vi "Game Engine.vi"(6 "UI Refs":T1, 10 "Dashboard":T2[](array[typedef]), 11 "SquareBattle in":refnum<class "SquareBattle.lvclass">) -> ()   [LabVIEW 2014, in "SquareBattle.lvclass"]
uses:
  SquareBattle.lvclass
  Dashboard.ctl
  UI Refs.ctl
  Runner Cluster.ctl
  Runner/Runner.lvclass
  Move State Cluster.ctl
  Action Enum.ctl
  Move Queue Element Cluster.ctl
  Direction Enum.ctl
  SquareBattle.lvclass/SquareBattle.ctl
  Runner/Runner.lvclass/Runner.ctl
panel:
  # "NOTICE - YOU MUST NOT REMOVE THIS NOTICE. PER THE FOLLOWING LICENSE, YOU MAY REPRODUCE THIS SOFTWARE PROVIDED YOU FOLLOW THE TERMS\nOF THE LICENSE.\n\n---BEGIN BSD LICENSE (http://opensource.org/licenses/BSD-2-Clause)---\nCopyright (c) 2015, Endigit, Inc. <robert@endigit.com>\nAll rights reserved.\n\nRedistribution and use in source and binary forms, with or without modification, are permitted provided that the following conditions are met:\n\n1. Redistributions of source code must retain the above copyright notice, this list of conditions and the following disclaimer.\n\n2. Redistributions in binary form must reproduce the above copyright notice, this list of conditions and the following disclaimer in the documentation and/or other \nmaterials provided with the distribution.\n\nTHIS SOFTWARE IS PROVIDED BY THE COPYRIGHT HOLDERS AND CONTRIBUTORS \"AS IS\" AND ANY EXPRESS OR IMPLIED WARRANTIES, INCLUDING, BUT NOT \nLIMITED TO, THE IMPLIED WARRANTIES OF MERCHANTABILITY AND FITNESS FOR A PARTICULAR PURPOSE ARE DISCLAIMED. IN NO EVENT SHALL THE COPYRIGHT \nHOLDER OR CONTRIBUTORS BE LIABLE FOR ANY DIRECT, INDIRECT, INCIDENTAL, SPECIAL, EXEMPLARY, OR CONSEQUENTIAL DAMAGES (INCLUDING, BUT NOT \nLIMITED TO, PROCUREMENT OF SUBSTITUTE GOODS OR SERVICES; LOSS OF USE, DATA, OR PROFITS; OR BUSINESS INTERRUPTION) HOWEVER CAUSED AND ON \nANY THEORY OF LIABILITY, WHETHER IN CONTRACT, STRICT LIABILITY, OR TORT (INCLUDING NEGLIGENCE OR OTHERWISE) ARISING IN ANY WAY OUT OF THE USE \nOF THIS SOFTWARE, EVEN IF ADVISED OF THE POSSIBILITY OF SUCH DAMAGE.\n---END BSD LICENSE---"
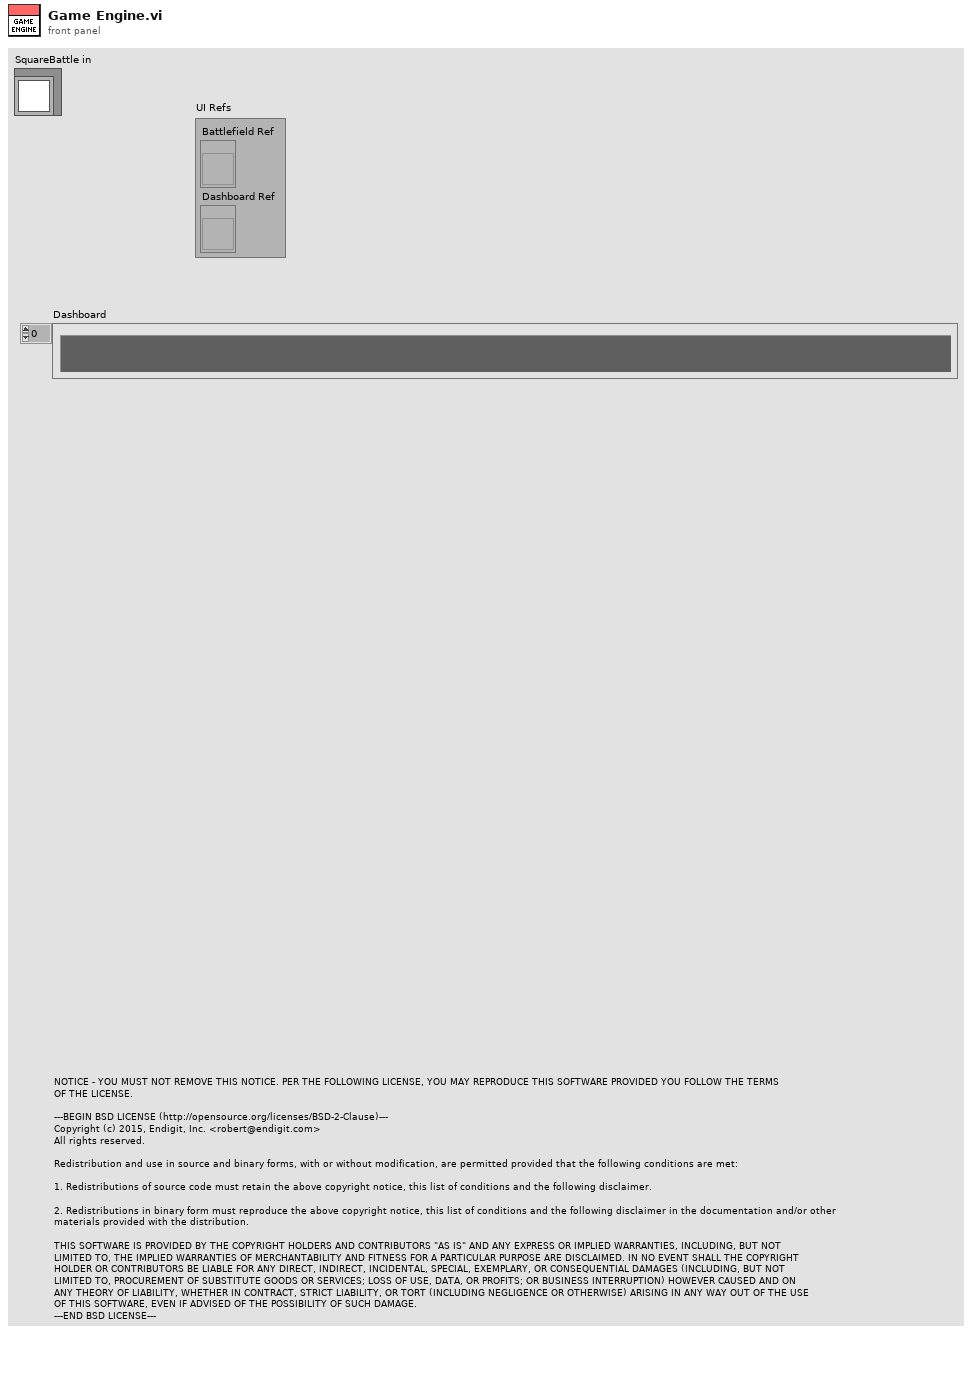
[diagram p1: front panel]
types:
  T1 = typedef "SquareBattle.lvclass/UI Refs.ctl" = cluster{"Battlefield Ref":refnum<vi>, "Dashboard Ref":refnum<vi>}
  T2 = typedef "SquareBattle.lvclass/Dashboard.ctl" = cluster{"Color":u32, "Player":string, "Status":string}
  T3 = typedef "SquareBattle.lvclass/Move Queue Element Cluster.ctl" = cluster{"Team Idx":i32, "NextTurn":u32, "YX Pos":string, "s Taken":dbl, "RunnerRef":refnum<data-value>, "Action":T4, "Direction":T5, "Player#":i32, "Replicated":refnum<class "Runner.lvclass">}
  T4 = typedef "SquareBattle.lvclass/Action Enum.ctl" = enum16{"Wait", "Move", "Attack", "Replicate"}
  T5 = typedef "SquareBattle.lvclass/Direction Enum.ctl" = enum16{"NW", "N", "NE", "E", "SE", "S", "SW", "W"}
  T6 = typedef "SquareBattle.lvclass/Move State Cluster.ctl" = cluster{"InPlayPos Dict":variant}
  T7 = typedef "SquareBattle.lvclass/Runner Cluster.ctl" = cluster{"Attacked?":bool, "DVR":refnum<data-value>, "Team":i32, "Player":i32, "Wait":u32}
  T8 = typedef "SquareBattle.lvclass/Player Info.ctl" = cluster{"Name":string, "Color Box":u32, "Gloat Phrase":string}
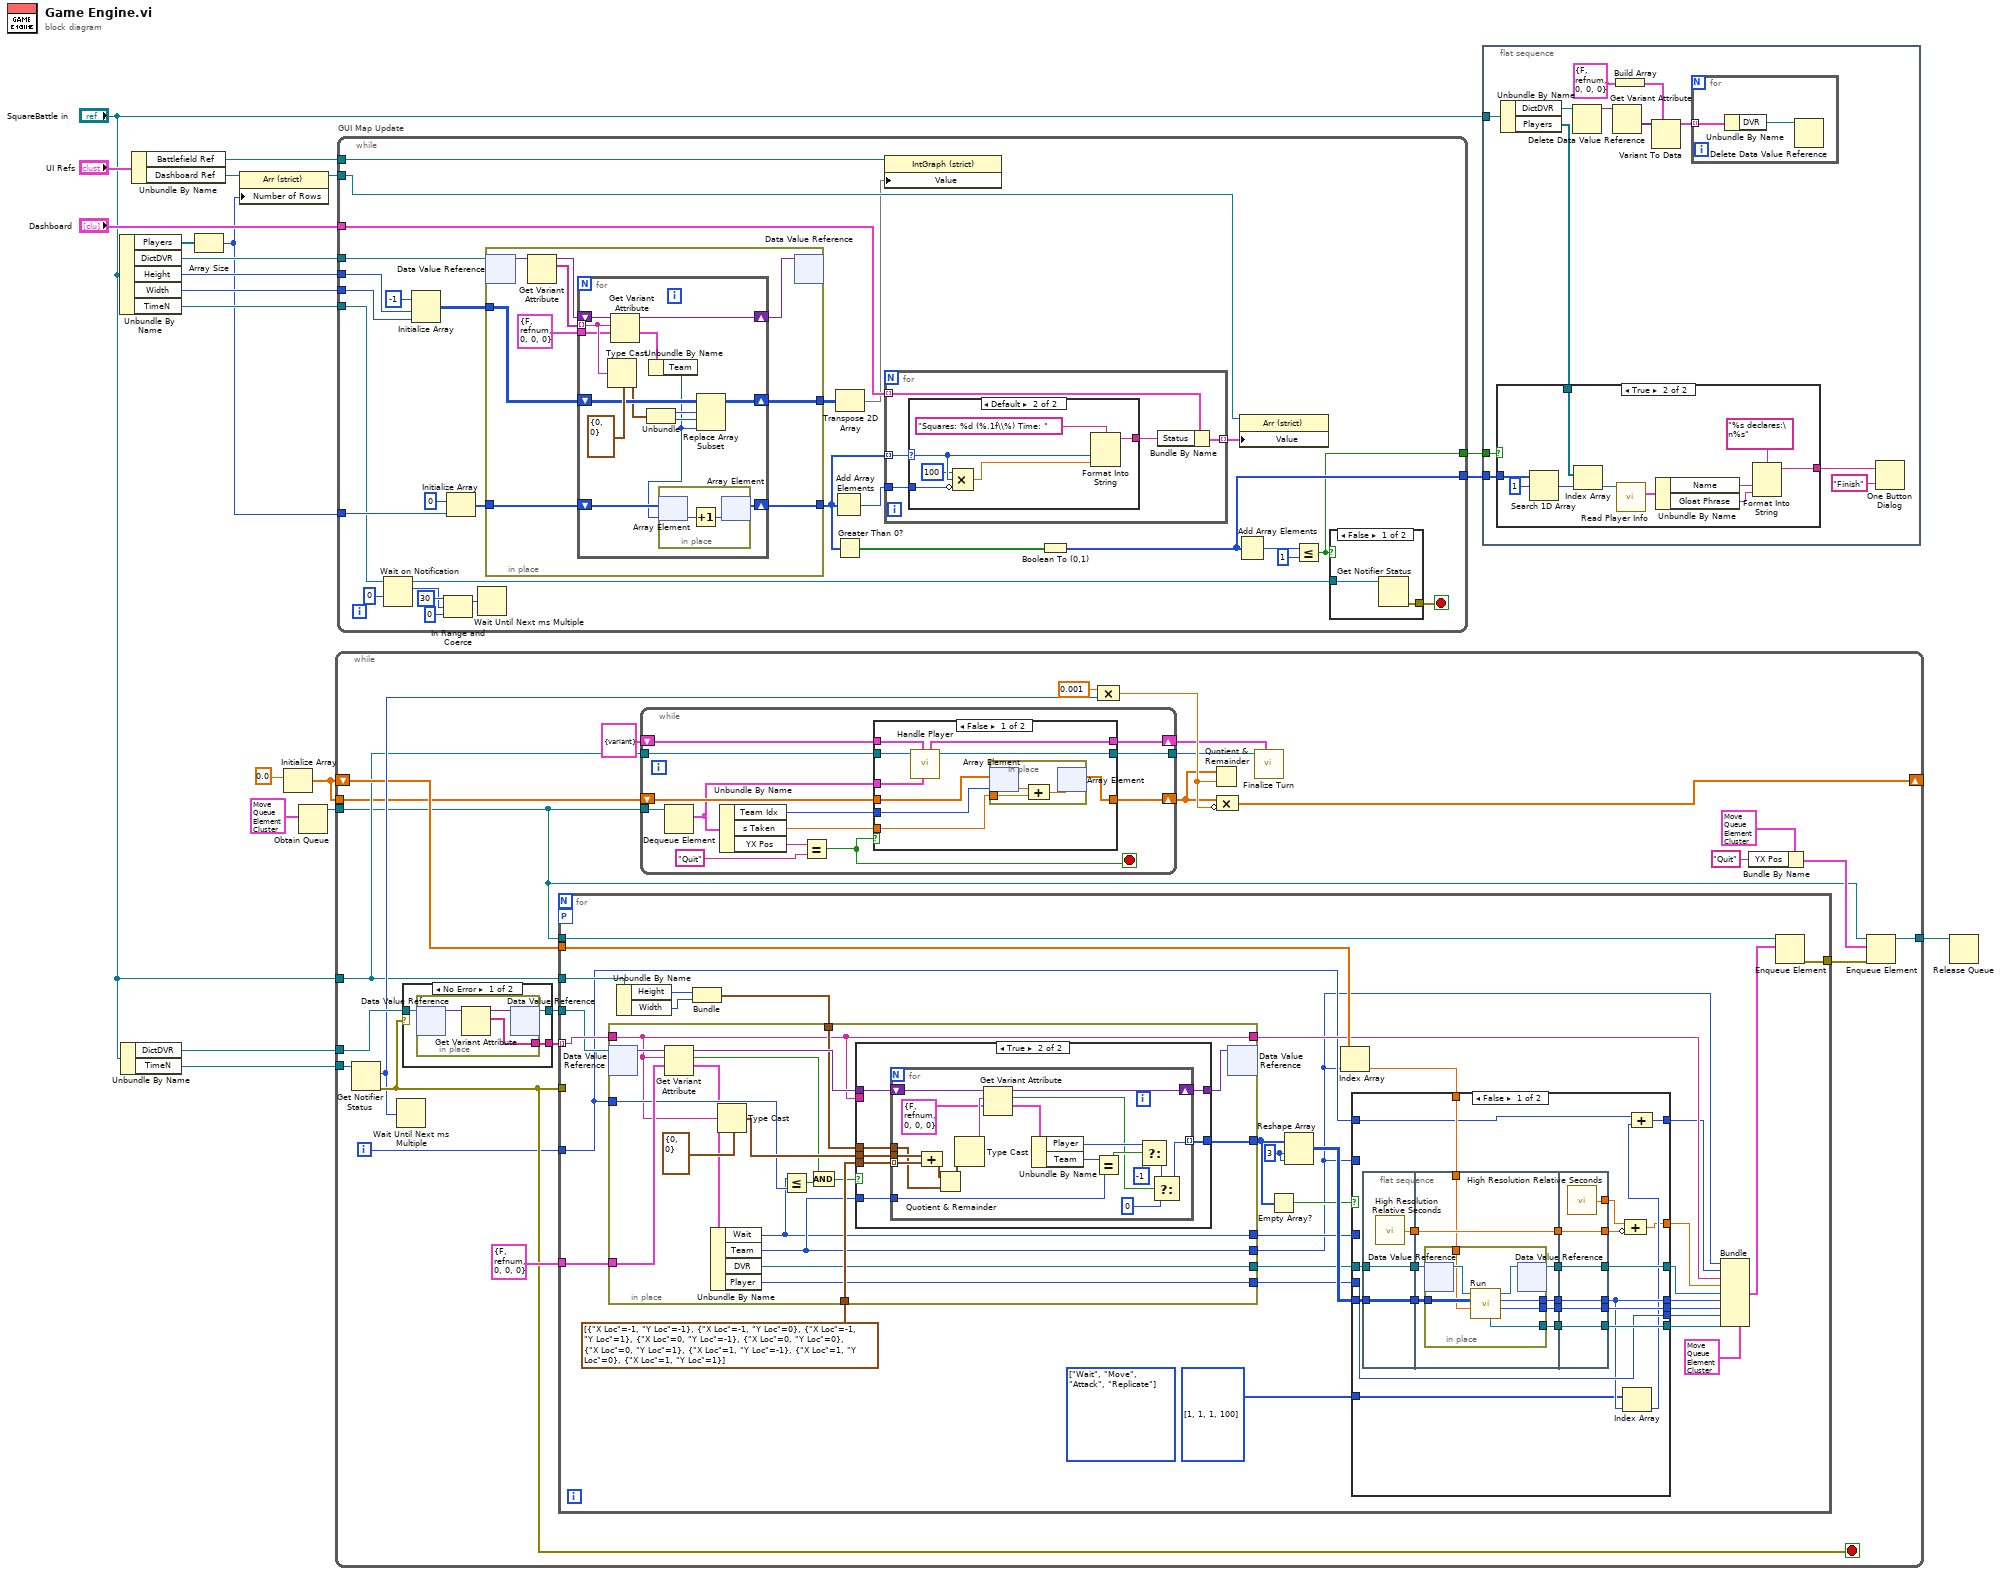
[diagram p0: block diagram]
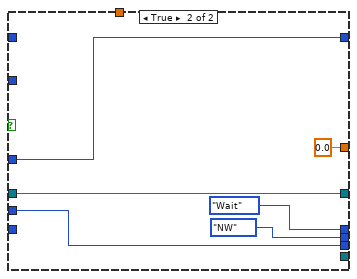
[diagram p4: hidden frame]
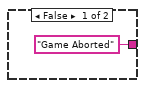
[diagram p6: hidden frame]
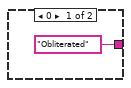
[diagram p7: hidden frame]
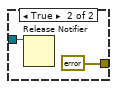
[diagram p8: hidden frame]
diagram:
  n1 = Unbundle By Name("SquareBattle in") -> ("Players"=w14:refnum<class "Runner.lvclass">[], "DictDVR"=w13:refnum<data-value>, "Height"=w12:i32, "Width"=w11:i32, "TimeN"=w10:refnum<notifier>)
  n2 = Unbundle By Name("SquareBattle in") -> ("DictDVR"=w8:refnum<data-value>, "TimeN"=w7:refnum<notifier>)
  n3 = Unbundle By Name("UI Refs") -> ("Battlefield Ref"=w19:refnum<vi>, "Dashboard Ref"=w16:refnum<vi>)
  n4 = Array Size(array=w14) -> (size(s)=w9:i32)
  n5 = property on="Property Node" class="Arr (strict)"(reference=w16, "Number of Rows"=w9) -> (reference out=w15:refnum<vi>)  [unwired: 1 in, 1 out]
  n6 = Initialize Array(0.0) -> (w4:dbl[])  [unwired: 1 in]
  n7 = Obtain Queue(element data type=T3 {"Team Idx"=0, "NextTurn"=0, "YX Pos"="", "s Taken"=0.0, "RunnerRef"=refnum, "Action"=enum."Wait", "Direction"=enum."NW", "Player#"=0, "Replicated"=refnum} ("Move Queue Element")) -> (queue out=w5:refnum<queue>)  [unwired: 4 in, 2 out]
  n8 = while {
    tunnel: w8 -> [w45]
    tunnel: w7 -> [w41]
    tunnel: "SquareBattle in" -> [w33]
    shift-right: [w36] -> _
    shift-left: w4 -> [w34]
    tunnel: w5 -> [w22]
    tunnel: w4 -> [w31]
    tunnel: [w27] -> w3
    i -> [w39]
    stop <- w40 stop-if-true
    n9 = Get Notifier Status(notifier=w41) -> (current notification=w38:u32, error out=w40:errorcluster)  [unwired: 1 in, 3 out]
    n10 = Wait Until Next ms Multiple(millisecond multiple=w38) -> ()  [unwired: 1 out]
    n11 = case shown="No Error" w40 {
      tunnel: w45 -> [w76 w80]
      tunnel: [w75 _] -> w44
      tunnel: [w74 w80] -> w43
      frame No Error {
        n12 = in-place {
          in-place-border: [w77] -> w75
          n13 = in-place-dvr #1(w76) -> (w79:variant)  [unwired: 1 out]
          n14 = Get Variant Attribute(Variant=w79) -> (duplicate Variant=w78:variant, names=w77:string[])  [unwired: 3 in, 2 out]
          n15 = in-place-dvr #1(w78) -> (w74:refnum<data-value>)  [unwired: 1 out]
        }
      }
      frame Error {
      }
    }
    n16 = for {
      tunnel: w39 -> [w90]
      tunnel: w40 -> [_]
      tunnel: w33 -> [w112]
      tunnel: w44 -> [w111] mode=indexing
      tunnel: w43 -> [w100]
      tunnel: T7 {"Attacked?"=FALSE, "DVR"=refnum, "Team"=0, "Player"=0, "Wait"=0} ("Cluster") -> [w110]
      tunnel: w34 -> [w99]
      workers-P: _ -> [_]
      tunnel: w22 -> [w84]
      tunnel: [w81] -> w23
      (unwired) T4[] [enum."Wait", enum."Move", enum."Attack", enum."Replicate"] items=["Wait", "Move", "Attack", "Replicate"]
      w107 = 3 ("dimension size")
      n17 = Unbundle By Name(w112) -> ("Height"=w106:i32, "Width"=w105:i32)
      n18 = Bundle("Height"=w106, "Width"=w105) -> (w104:cluster{"Height":i32, "Width":i32})  [unwired: 1 in]
      n19 = in-place {
        in-place-border: cluster{"X Loc":i32, "Y Loc":i32}[] [{"X Loc"=-1, "Y Loc"=-1}, {"X Loc"=-1, "Y Loc"=0}, {"X Loc"=-1, "Y Loc"=1}, {"X Loc"=0, "Y Loc"=-1}, {"X Loc"=0, "Y Loc"=0}, {"X Loc"=0, "Y Loc"=1}, {"X Loc"=1, "Y Loc"=-1}, {"X Loc"=1, "Y Loc"=0}, {"X Loc"=1, "Y Loc"=1}] -> [w184]
        in-place-border: [w183] -> w103
        in-place-border: w111 -> [w170]
        in-place-border: w110 -> [w181]
        in-place-border: w90 -> [w178]
        in-place-border: w104 -> [w174]
        in-place-border: [w171] -> w101
        in-place-border: [w170] -> w94
        in-place-border: [w168] -> w86
        in-place-border: [w167] -> w92
        in-place-border: [w166] -> w88
        n20 = in-place-dvr #2(w100) -> (w182:variant)  [unwired: 1 out]
        n21 = Get Variant Attribute(Variant=w182, name=w170, default value (empty Variant)=w181) -> (duplicate Variant=w177:variant, found=w173:bool, value=w172:T7)  [unwired: 1 in, 1 out]
        n22 = Unbundle By Name(w172) -> ("Wait"=w166:u32, "Team"=w168:i32, "DVR"=w171:refnum<data-value>, "Player"=w167:i32)
        n23 = Type Cast(type=cluster{"Y":i32, "X":i32} {"Y"=0, "X"=0}, x=w170) -> (*(type *) &x=w179:cluster{"Y":i32, "X":i32})
        n24 = Less Or Equal?(x=w166, y=w178) -> (x <= y?=w176:bool)
        n25 = Compound Arithmetic op=AND(w173, w176) -> (w169:bool)
        n26 = case shown="True" w169 {
          tunnel: w184 -> [_ w192]
          tunnel: [_ w191] -> w183
          tunnel: w168 -> [_ w190]
          tunnel: w179 -> [_ w189]
          tunnel: w177 -> [w185 w188]
          tunnel: [w185 w187] -> w175
          tunnel: w174 -> [_ w186]
          tunnel: w170 -> [_ _]
          frame False {
          }
          frame True {
            n27 = for {
              tunnel: w189 -> [w211]
              tunnel: w186 -> [w208]
              tunnel: w192 -> [w210] mode=indexing
              tunnel: [w206] -> w191 mode=indexing
              tunnel: w190 -> [w200]
              shift-right: [w193] -> w187
              shift-left: w188 -> [w198]
              n28 = Compound Arithmetic op=ADD(w211, w210) -> (w209:cluster{i32, i32})
              n29 = Quotient & Remainder(x=w209, y=w208) -> (x-y*floor(x/y)=w199:cluster{i32, i32})  [unwired: 1 out]
              n30 = Type Cast(x=w199) -> (*(type *) &x=w197:string)  [unwired: 1 in]
              n31 = Get Variant Attribute(Variant=w198, name=w197, default value (empty Variant)=T7 {"Attacked?"=FALSE, "DVR"=refnum, "Team"=0, "Player"=0, "Wait"=0} ("Cluster")) -> (duplicate Variant=w193:variant, found=w194:bool, value=w195:T7)  [unwired: 1 in, 1 out]
              n32 = Unbundle By Name(w195) -> ("Player"=w204:i32, "Team"=w202:i32)
              n33 = Equal?(x=w202, y=w200) -> (x = y?=w201:bool)
              n34 = Select(t=w204, s=w201, f=-1) -> (s? t:f=w205:i32)
              n35 = Select(t=w205, s=w194, f=0) -> (s? t:f=w206:i32)
            }
          }
        }
        n36 = in-place-dvr #2(w175) -> ()  [unwired: 2 out]
      }
      n37 = Empty Array?(array=w103) -> (empty?=w102:bool)
      n38 = Reshape Array(w103, w107, w107) -> (w108:i32[][])
      n39 = Index Array(array=w99, index=w86) -> (element=w95:dbl)
      n40 = case shown="False" w102 {
        tunnel: w101 -> [w128 w163]
        tunnel: w108 -> [w127 _]
        tunnel: [w116 Action_Enum."Wait" ("Action")] -> w98
        tunnel: [w124 Direction_Enum."NW" ("Direction")] -> w97
        tunnel: [w123 _] -> w96
        tunnel: w86 -> [_ _]
        tunnel: w95 -> [w122 _]
        tunnel: [w121 w163] -> w93
        tunnel: w92 -> [w119 w162]
        tunnel: [w119 w162] -> w91
        tunnel: w90 -> [w118 _]
        tunnel: [w117 w161] -> w87
        tunnel: u32[] [1, 1, 1, 100] -> [w115 _]
        tunnel: w88 -> [_ w161]
        tunnel: [w113 0.0] -> w85
        frame False {
          n41 = flat-sequence {
            tunnel: w127 -> [w137]
            tunnel: w128 -> [w138]
            tunnel: [w138] -> w135
            tunnel: [w137] -> w134
            tunnel: [w136] -> w133
            tunnel: [w144] -> w132
            tunnel: [w143] -> w131
            tunnel: [w142] -> w130
            tunnel: w135 -> [w146]
            tunnel: w134 -> [w145]
            tunnel: w133 -> [w141]
            tunnel: [w141] -> w129
            tunnel: w122 -> [w140]
            tunnel: [w139] -> w120
            tunnel: [w157] -> w123
            tunnel: [w158] -> w124
            tunnel: [w159] -> w116
            tunnel: w132 -> [w159]
            tunnel: w131 -> [w158]
            tunnel: w130 -> [w157]
            tunnel: [w156] -> w125
            tunnel: w129 -> [w156]
            tunnel: [w155] -> w126
            tunnel: [w154] -> w121
            tunnel: w120 -> [w154]
            frame #0 {
              n42 = call <vilib>:"High Resolution Relative Seconds.vi"() -> ("relative seconds"=w136:dbl)
            }
            frame #1 {
              n43 = in-place {
                in-place-border: w145 -> [w151]
                in-place-border: [w150] -> w144
                in-place-border: [w149] -> w143
                in-place-border: [w148] -> w142
                in-place-border: w140 -> [w147]
                n44 = in-place-dvr #3(w146) -> (w153:refnum<class "Runner.lvclass">)  [unwired: 1 out]
                n45 = call-dynamic "Run.vi"("Time Ratio used"=w147, "Maze (0: Empty, -1: Enemy. >0: Teammate"=w151, "Runner in"=w153) -> ("Direction"=w149:T5, "Action"=w150:T4, "Runner out"=w152:refnum<class "Runner.lvclass">, "Replicated"=w148:refnum<class "Runner.lvclass">)  [unwired: 4 in, 1 out]
                n46 = in-place-dvr #3(w152) -> (w139:refnum<data-value>)  [unwired: 1 out]
              }
            }
            frame #2 {
              n47 = call <vilib>:"High Resolution Relative Seconds.vi"() -> ("relative seconds"=w155:dbl)
            }
          }
          n48 = Index Array(array=w115, index=w116) -> (element=w114:u32)
          n49 = Compound Arithmetic op=ADD(w126, invert w125) -> (w113:dbl)
          n50 = Compound Arithmetic op=ADD(w118, w114) -> (w117:u32)
        }
        frame True {
        }
      }
      n51 = Bundle(cluster=T3 {"Team Idx"=0, "NextTurn"=0, "YX Pos"="", "s Taken"=0.0, "RunnerRef"=refnum, "Action"=enum."Wait", "Direction"=enum."NW", "Player#"=0, "Replicated"=refnum} ("Move Queue Element"), "Team Idx"=w86, "NextTurn"=w87, "YX Pos"=w94, "s Taken"=w85, "RunnerRef"=w93, "Action"=w98, "Direction"=w97, "Player#"=w91, "Replicated"=w96) -> (w83:T3)
      n52 = Enqueue Element(queue=w84, element=w83) -> (error out=w81:errorcluster)  [unwired: 2 in, 2 out]
    }
    n53 = while {
      tunnel: w22 -> [w55]
      tunnel: w33 -> [w56]
      shift-right: [w57] -> w28
      shift-left: T6 {"InPlayPos Dict"=variant(i32[] [])} ("Cluster") -> [w58]
      shift-right: [w53] -> w30
      shift-left: w31 -> [w54]
      tunnel: [w50] -> w29
      stop <- w46 stop-if-true
      n54 = Dequeue Element(queue=w55) -> (element=w49:T3)  [unwired: 2 in, 3 out]
      n55 = Unbundle By Name(w49) -> ("Team Idx"=w52:i32, "s Taken"=w51:dbl, "YX Pos"=w48:string)
      n56 = Equal?(x=w48, y="Quit") -> (x = y?=w46:bool)
      n57 = case shown="False" w46 {
        tunnel: w58 -> [w67 w73]
        tunnel: [w66 w73] -> w57
        tunnel: w56 -> [w65 w72]
        tunnel: w54 -> [w64 w71]
        tunnel: [w63 w71] -> w53
        tunnel: w52 -> [w62 _]
        tunnel: w51 -> [w61 _]
        tunnel: [w60 w72] -> w50
        tunnel: w49 -> [w59 _]
        frame False {
          n58 = call "Handle Player.vi"("Move Queue Element"=w59, "Move in"=w67, "Maze 2.0 in"=w65) -> ("Maze 2.0 out"=w60:refnum<class "SquareBattle.lvclass">, "Move out"=w66:T6)  [unwired: 7 in]
          n59 = in-place {
            in-place-border: w61 -> [w68]
            n60 = in-place-array #4(w64, w62) -> (w70:dbl)
            n61 = Compound Arithmetic op=ADD(w70, w68) -> (w69:dbl)
            n62 = in-place-array #4(w69) -> (w63:dbl[])  [unwired: 1 out]
          }
        }
        frame True {
        }
      }
    }
    n63 = Compound Arithmetic op=MULTIPLY(0.001, w38) -> (w35:dbl)
    n64 = Quotient & Remainder(x=w30, y=w35) -> ()  [unwired: 2 out]
    n65 = Compound Arithmetic op=MULTIPLY(w30, invert w35) -> (w36:dbl[])
    n66 = call "Finalize Turn.vi"("Move State"=w28, "Maze 2.0 in"=w29) -> ()  [unwired: 8 in, 2 out]
    n67 = Bundle By Name(cluster=T3 {"Team Idx"=0, "NextTurn"=0, "YX Pos"="", "s Taken"=0.0, "RunnerRef"=refnum, "Action"=enum."Wait", "Direction"=enum."NW", "Player#"=0, "Replicated"=refnum} ("Move Queue Element"), "YX Pos"="Quit") -> (w24:T3)
    n68 = Enqueue Element(queue=w22, element=w24, error in (no error)=w23) -> (queue out=w27:refnum<queue>)  [unwired: 1 in, 2 out]
  }
  n69 = while "GUI Map Update" {
    tunnel: w9 -> [w235]
    tunnel: "Dashboard" -> [w230]
    tunnel: w15 -> [w226]
    tunnel: w19 -> [w224]
    tunnel: [w223] -> w18
    tunnel: [w222] -> w17
    tunnel: w13 -> [w215]
    tunnel: w12 -> [w214]
    tunnel: w11 -> [w213]
    tunnel: w10 -> [w212]
    stop <- w232 stop-if-true
    n70 = Wait on Notification(notifier=w212, timeout in ms (-1)=0) -> (notifier out=w218:refnum<notifier>, notification=w216:u32)  [unwired: 2 in, 2 out]
    n71 = Initialize Array(-1, w214, w213) -> (w236:i32[][])
    n72 = In Range and Coerce(upper limit=u32 30 ("millisecond multiple"), x=w216, lower limit=u32 0) -> (coerced(x)=w221:u32)  [unwired: 1 out]
    n73 = Initialize Array(0 ("element"), w235) -> (w233:i32[])
    n74 = Wait Until Next ms Multiple(millisecond multiple=w221) -> ()  [unwired: 1 out]
    n75 = in-place {
      in-place-border: [w265] -> w231
      in-place-border: w236 -> [w262]
      in-place-border: w233 -> [w258]
      in-place-border: [w257] -> w229
      n76 = in-place-dvr #5(w215) -> (w264:variant)  [unwired: 1 out]
      n77 = Get Variant Attribute(Variant=w264) -> (duplicate Variant=w261:variant, names=w263:string[])  [unwired: 3 in, 2 out]
      n78 = for {
        tunnel: w263 -> [w277] mode=indexing
        shift-right: [w273] -> w265
        shift-left: w262 -> [w274]
        shift-right: [w276] -> w260
        shift-left: w261 -> [w279]
        tunnel: T7 {"Attacked?"=FALSE, "DVR"=refnum, "Team"=0, "Player"=0, "Wait"=0} ("Cluster") -> [w275]
        shift-right: [w268] -> w257
        shift-left: w258 -> [w267]
        n79 = Type Cast(type=cluster{"Y":i32, "X":i32} {"Y"=0, "X"=0}, x=w277) -> (*(type *) &x=w272:cluster{"Y":i32, "X":i32})
        n80 = Get Variant Attribute(Variant=w279, name=w277, default value (empty Variant)=w275) -> (duplicate Variant=w276:variant, value=w269:T7)  [unwired: 1 in, 2 out]
        n81 = Unbundle(w272) -> ("Y"=w271:i32, "X"=w270:i32)
        n82 = Unbundle By Name(w269) -> ("Team"=w266:i32)
        n83 = in-place {
          n84 = in-place-array #6(w267, w266) -> (w281:i32)
          n85 = Increment(x=w281) -> (x+1=w280:i32)
          n86 = in-place-array #6(w280) -> (w268:i32[])  [unwired: 1 out]
        }
        n87 = Replace Array Subset(array=w274, new element=w266, index (row)=w271, index (col)=w270) -> (w273:i32[][])
      }
      n88 = in-place-dvr #5(w260) -> ()  [unwired: 2 out]
    }
    n89 = Add Array Elements(numeric array=w229) -> (sum=w228:i32)
    n90 = Greater Than 0?(x=w229) -> (x > 0?=w240:bool[])
    n91 = Transpose 2D Array(2D array=w231) -> (transposed array=w225:i32[][])
    n92 = property on="Property Node" class="IntGraph (strict)"(reference=w224, "Value"=w225) -> ()  [unwired: 1 in, 2 out]
    n93 = for {
      tunnel: w230 -> [w245] mode=indexing
      tunnel: [w244] -> w227 mode=indexing
      tunnel: w229 -> [w242] mode=indexing
      tunnel: w228 -> [w241]
      n94 = case shown="Default" w242 {
        selector: w242 -> [_ w249]
        tunnel: ["Obliterated" w251] -> w243
        tunnel: w241 -> [_ w248]
        frame 0 {
        }
        frame Default {
          n95 = Compound Arithmetic op=MULTIPLY(100 ("value"), w249, invert w248) -> (w250:dbl)
          n96 = Format Into String(format string="Squares: %d (%.1f\\%) Time: ", w249, w250) -> (resulting string=w251:string)  [unwired: 2 in, 1 out]
        }
      }
      n97 = Bundle By Name(cluster=w245, "Status"=w243) -> (w244:T2)
    }
    n98 = Boolean To (0,1)(Boolean=w240) -> (0, 1=w223:i16[])
    n99 = Add Array Elements(numeric array=w223) -> (sum=w239:i16)
    n100 = property on="Property Node" class="Arr (strict)"(reference=w226, "Value"=w227) -> ()  [unwired: 1 in, 2 out]
    n101 = Less Or Equal?(x=w239, y=i16 1) -> (x <= y?=w222:bool)
    n102 = case shown="False" w222 {
      tunnel: w218 -> [w254 w256]
      tunnel: [w253 errorcluster {"status"=TRUE, "code"=0, "source"=""} ("error out")] -> w232
      frame False {
        n103 = Get Notifier Status(notifier=w254) -> (error out=w253:errorcluster)  [unwired: 1 in, 4 out]
      }
      frame True {
        n104 = Release Notifier(notifier=w256) -> ()  [unwired: 2 in, 3 out]
      }
    }
  }
  n105 = flat-sequence {
    tunnel: "SquareBattle in" -> [w291]
    tunnel: w18 -> [w284]
    tunnel: w17 -> [w282]
    frame #0 {
      n106 = Unbundle By Name(w291) -> ("DictDVR"=w293:refnum<data-value>, "Players"=w283:refnum<class "Runner.lvclass">[])
      n107 = case shown="True" w282 {
        tunnel: ["Game Aborted" w303] -> w290
        tunnel: w284 -> [_ w302]
        tunnel: w283 -> [_ w299]
        frame False {
        }
        frame True {
          n108 = Search 1D Array(1D array=w302, element=i16 1) -> (index of element=w300:i32)  [unwired: 1 in]
          n109 = Index Array(array=w299, index=w300) -> (element=w298:refnum<class "Runner.lvclass">)
          n110 = call "Read Player Info.vi"("Runner in"=w298) -> ("Player Info"=w297:T8)  [unwired: 8 in, 2 out]
          n111 = Unbundle By Name(w297) -> ("Name"=w296:string, "Gloat Phrase"=w295:string)
          n112 = Format Into String(format string="%s declares:\n%s", w296, w295) -> (resulting string=w303:string)  [unwired: 2 in, 1 out]
        }
      }
      n113 = Delete Data Value Reference(data value reference=w293) -> (data value=w292:variant)  [unwired: 1 in, 1 out]
      n114 = Get Variant Attribute(Variant=w292) -> (values=w287:variant[])  [unwired: 3 in, 3 out]
      n115 = Build Array(T7 {"Attacked?"=FALSE, "DVR"=refnum, "Team"=0, "Player"=0, "Wait"=0} ("Cluster")) -> (w286:T7[])
      n116 = Variant To Data(type=w286, Variant=w287) -> (data=w285:T7[])  [unwired: 1 in, 1 out]
      n117 = for {
        tunnel: w285 -> [w305] mode=indexing
        n118 = Unbundle By Name(w305) -> ("DVR"=w306:refnum<data-value>)
        n119 = Delete Data Value Reference(data value reference=w306) -> ()  [unwired: 1 in, 2 out]
      }
      n120 = One Button Dialog(message=w290, button name ("OK")="Finish") -> ()  [unwired: 1 out]
    }
  }
  n121 = Release Queue(queue=w3) -> ()  [unwired: 2 in, 3 out]
